vi "Set Table Control Ref.vi"(8 "error in (no error)":errorcluster, 10 "Table Control":refnum<vi>, 11 "List_UI in":refnum<class "List_UI.lvclass">) -> (0 "error out":errorcluster, 3 "List_UI out":refnum<class "List_UI.lvclass">)   [LabVIEW 2015, in "List_UI.lvclass"]
uses:
  List_UI.lvclass
  List_UI.lvclass/List_UI.ctl
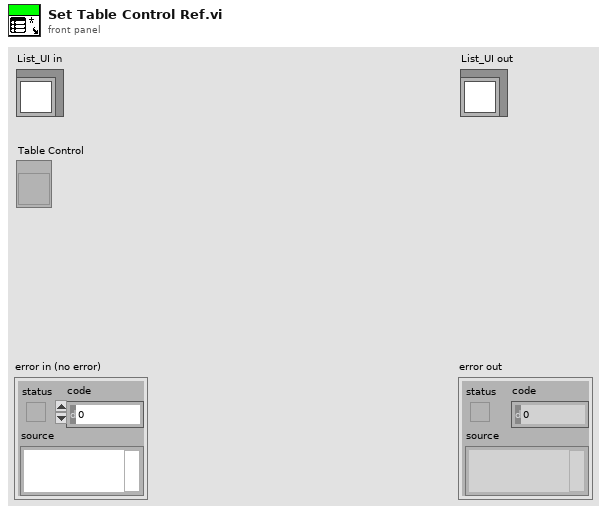
[diagram p1: front panel]
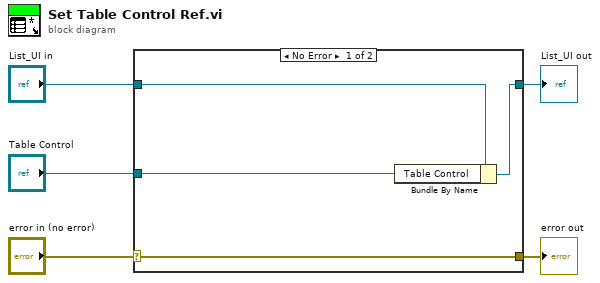
[diagram p0: block diagram]
diagram:
  n1 = case shown="No Error" "error in (no error)" {
    selector: "error in (no error)" -> [w9 w10]
    tunnel: [w9 w10] -> w4
    tunnel: [w7 w11] -> w2
    tunnel: "List_UI in" -> [w8 w11]
    tunnel: "Table Control" -> [w6 _]
    frame No Error {
      n2 = Bundle By Name(cluster=w8, "Table Control"=w6) -> (w7:refnum<class "List_UI.lvclass">)
    }
    frame Error {
    }
  }
  "error out" <- w4
  "List_UI out" <- w2
